vi "Radau5_Nan and Inf Check.vi"(7 "Width":i32, 8 "Input Array Y'":dbl[](array[numeric]), 9 "Input Array Y":dbl[](array[numeric]), 10 "Time Index":i32, 11 "SubIndex":i32) -> (0 "error out":errorcluster)   [LabVIEW 2017, in "NI_DAE.lvlib"]
uses:
  <vilib>/gmath/NI_DAE.lvlib
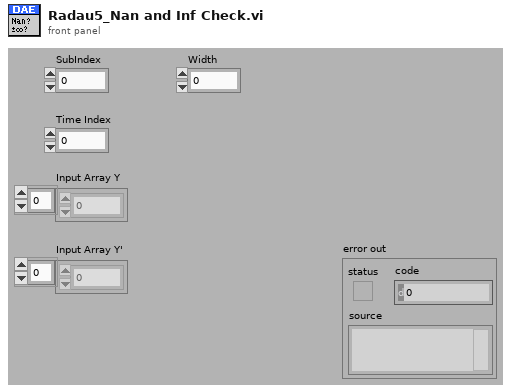
[diagram p1: front panel]
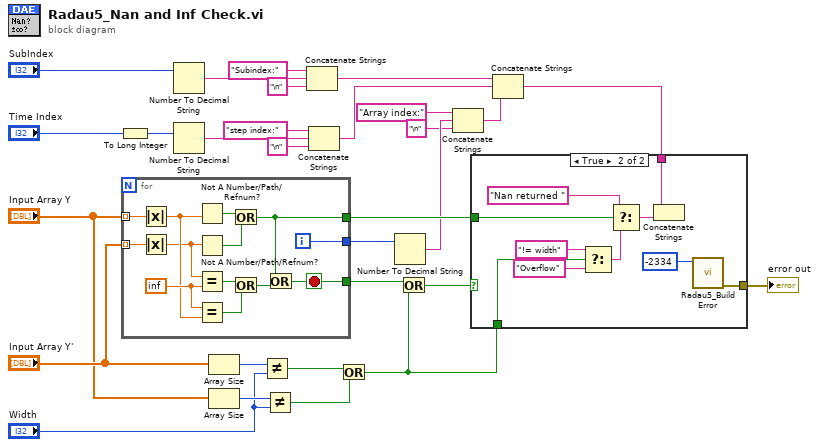
[diagram p0: block diagram]
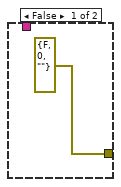
[diagram p2: hidden frame]
diagram:
  n1 = To Long Integer(number="Time Index") -> (32bit integer=w27:i32)
  n2 = for {
    tunnel: "Input Array Y" -> [w41] mode=indexing
    tunnel: "Input Array Y'" -> [w42] mode=indexing
    tunnel: [w38] -> w25
    tunnel: [w31] -> w29
    tunnel: [w30] -> w3
    i -> [w38]
    stop <- w30 stop-if-true
    w40 = inf
    n3 = Absolute Value(x=w41) -> (abs(x)=w39:dbl)
    n4 = Absolute Value(x=w42) -> (abs(x)=w35:dbl)
    n5 = Not A Number/Path/Refnum?(number/path/refnum=w39) -> (NaN/Path/Refnum?=w36:bool)
    n6 = Not A Number/Path/Refnum?(number/path/refnum=w35) -> (NaN/Path/Refnum?=w37:bool)
    n7 = Equal?(x=w35, y=w40) -> (x = y?=w34:bool)
    n8 = Equal?(x=w40, y=w39) -> (x = y?=w33:bool)
    n9 = Or(x=w36, y=w37) -> (x .or. y?=w31:bool)
    n10 = Or(x=w34, y=w33) -> (x .or. y?=w32:bool)
    n11 = Or(x=w31, y=w32) -> (x .or. y?=w30:bool)
  }
  n12 = Number To Decimal String(number="SubIndex") -> (decimal integer string=w23:string)  [unwired: 1 out]
  n13 = Number To Decimal String(number=w27) -> (decimal integer string=w20:string)  [unwired: 1 out]
  n14 = Array Size(array="Input Array Y'") -> (size(s)=w9:i32)
  n15 = Array Size(array="Input Array Y") -> (size(s)=w8:i32)
  n16 = Not Equal?(x=w9, y="Width") -> (x != y?=w5:bool)
  n17 = Not Equal?(x=w8, y="Width") -> (x != y?=w4:bool)
  n18 = Concatenate Strings("Subindex:", w23, "\n") -> (w15:string)
  n19 = Concatenate Strings("step index:", w20, "\n") -> (w14:string)
  n20 = Or(x=w5, y=w4) -> (x .or. y?=w2:bool)
  n21 = Number To Decimal String(number=w25) -> (decimal integer string=w17:string)  [unwired: 1 out]
  n22 = Or(x=w3, y=w2) -> (x .or. y?=w1:bool)
  n23 = Concatenate Strings("Array index:", w17, "\n") -> (w13:string)
  n24 = Concatenate Strings(w15, w14, w13) -> (w12:string)
  n25 = case shown="True" w1 {
    tunnel: w29 -> [_ w53]
    tunnel: w12 -> [_ w50]
    tunnel: [errorcluster {"status"=FALSE, "code"=0, "source"=""} ("Error Cluster") w45] -> w11
    tunnel: w2 -> [_ w49]
    frame False {
    }
    frame True {
      n26 = Select(t="!= width", s=w49, f="Overflow") -> (s? t:f=w46:string)
      n27 = Select(t="Nan returned ", s=w53, f=w46) -> (s? t:f=w51:string)
      n28 = Concatenate Strings(w50, w51) -> ()  [unwired: 1 out]
      n29 = call <vilib>:"Radau5_Build Error.vi"("error code"=-2334 ("error.code")) -> ("error out"=w45:errorcluster)  [unwired: 10 in]
    }
  }
  "error out" <- w11
